vi "QSM_Push to Queue.vi"(6 "Push to FRONT of Queue?":bool, 8 "error in (no error)":errorcluster, 9 "DATA.VARIANT":variant, 10 "QSM_RunStates":T2, 11 "QSMRef in":T1) -> (0 "error out":errorcluster, 3 "QSMRef out":T1)   [LabVIEW 2014, in "GUIUpdateQSM.lvlib"]
uses:
  GUIUpdateQSM.lvlib
  Controls/QSM_RunStates.ctl
  Controls/QSM_Reference.ctl
  Controls/QSM_DataType.ctl
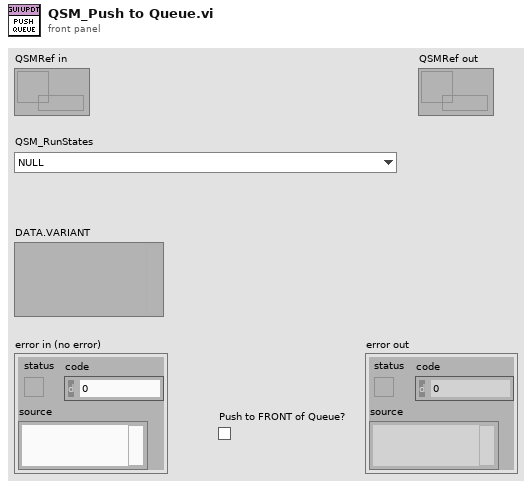
[diagram p1: front panel]
types:
  T1 = typedef "GUIUpdateQSM.lvlib/QSM_Reference.ctl" = refnum<queue>
  T2 = typedef "GUIUpdateQSM.lvlib/QSM_RunStates.ctl" = enum16{"NULL", "Sect01_Initialize-00_GROUP.ENQUEUE", "Sect01_Initialize-01_SetMainToDefault", "Sect01_Initialize-02_Clear Status Strings", "Sect02_UpdateUI-00_Enable Stop_ Disable Start", "Sect02_UpdateUI-01_Enable Start_Disable Stop", "Sect02_UpdateUI-02_Update Status String", "Sect02_UpdateUI-03_Clear XY-Graph", "Sect03-Open ROI  GUI", "Sect03-Close ROI GUI", "Sect99_EXIT-00_Group.Enqueue", "Sect99_EXIT-01_CloseReferences", "Sect99_EXIT-02_StopQSM"}
  T3 = typedef "GUIUpdateQSM.lvlib/QSM_DataType.ctl" = cluster{"QSM_RunStates":T2, "DATA.VARIANT":variant}
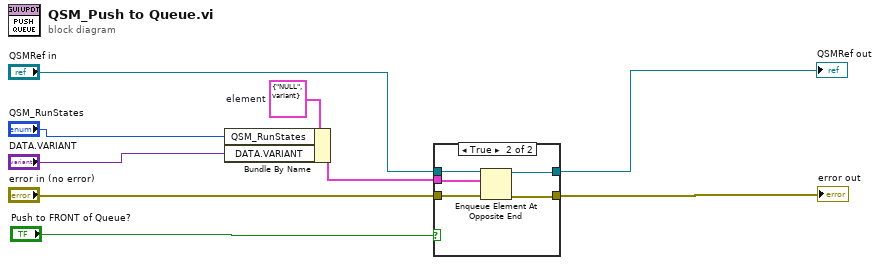
[diagram p0: block diagram]
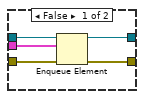
[diagram p2: hidden frame]
diagram:
  w7 = T3 {"QSM_RunStates"=enum."NULL", "DATA.VARIANT"=variant}  # element
  n1 = Bundle By Name(cluster=w7, "QSM_RunStates"="QSM_RunStates", "DATA.VARIANT"="DATA.VARIANT") -> (w3:T3)
  n2 = case shown="True" "Push to FRONT of Queue?" {
    tunnel: w3 -> [w14 w16]
    tunnel: [w13 w15] -> w1
    tunnel: "error in (no error)" -> [w12 w17]
    tunnel: "QSMRef in" -> [w11 w19]
    tunnel: [w10 w18] -> w2
    frame False {
      n3 = Enqueue Element(queue=w11, element=w14, error in (no error)=w12) -> (queue out=w10:T1, error out=w13:errorcluster)  [unwired: 1 in, 1 out]
    }
    frame True {
      n4 = Enqueue Element At Opposite End(queue=w19, element=w16, error in (no error)=w17) -> (queue out=w18:T1, error out=w15:errorcluster)  [unwired: 1 in, 1 out]
    }
  }
  "error out" <- w1
  "QSMRef out" <- w2
